vi "PID_controller_09.vi"() -> ()   [LabVIEW 2011]
panel:
  out "x/y":dbl
  out "fit":cluster{"element":dbl, "Value":dbl}[](array[cluster])
  out "err_avg":dbl
  out "Setpoint":string
  out "Angle (deg)":string
  in  "Ks":dbl
  out "dt(s)":dbl
  out "windup error":dbl
  out "tPrev":dbl
  out "target value":dbl
  out "error(t-t0)":cluster{dbl, "Value":dbl}[](array[cluster])
  out "error":dbl
  out "tStart(s)":dbl
  out "S00":dbl
  out "S10":dbl
  out "S20":dbl
  out "S11":dbl
  out "S01":dbl
  out "weight":dbl[](array[numeric])
  in  "# of points to watch":i32
  in  "tSmooth(s)":dbl=-1.0
  out "t0":dbl
  out "error(t)":cluster{dbl, "Value":dbl}[](array[cluster])
  out "error out":errorcluster
  out "first":bool=TRUE
  out "P (torr)":string
  out "XY Graph":T1(graph)
  out "current value":dbl
  in  "stop":bool
  in  "Period (s)":dbl
  out "dValue":dbl
  out "derivative":dbl
  out "integral":dbl
  out "Current angle (deg)":dbl
  in  "Kd":dbl
  in  "Ki":dbl
  in  "Kp":dbl
  out "Current P (torr)":dbl
  in  "Set Point (torr)":dbl
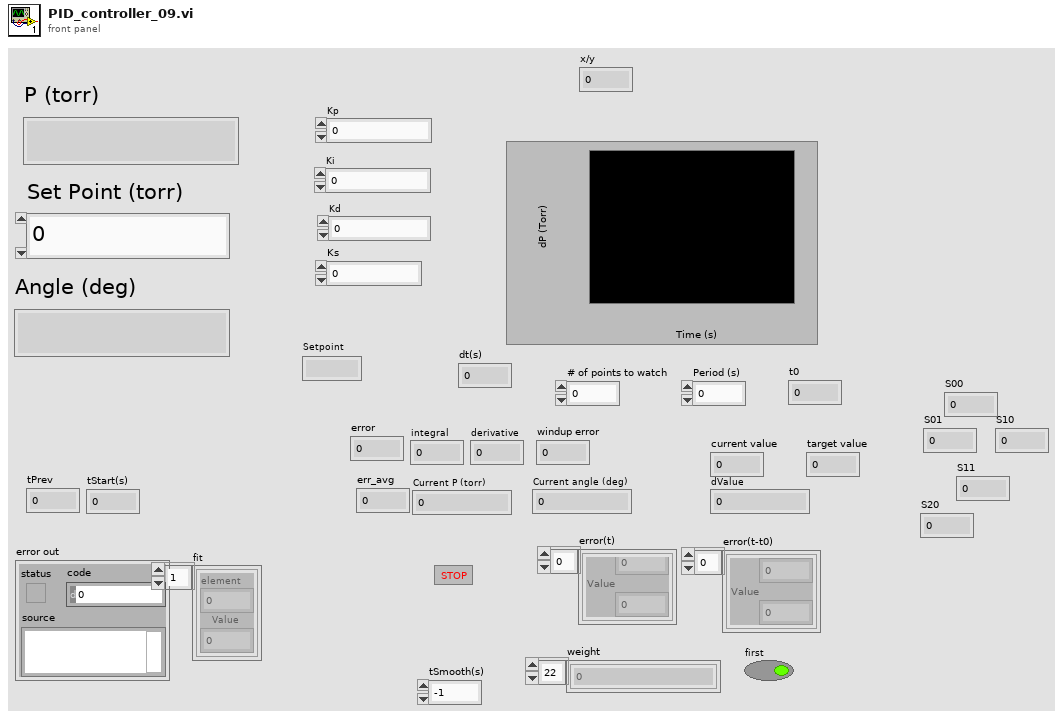
[diagram p1: front panel]
types:
  T1 = cluster{"Value":cluster{"element":dbl, "Value":dbl}[]}[]
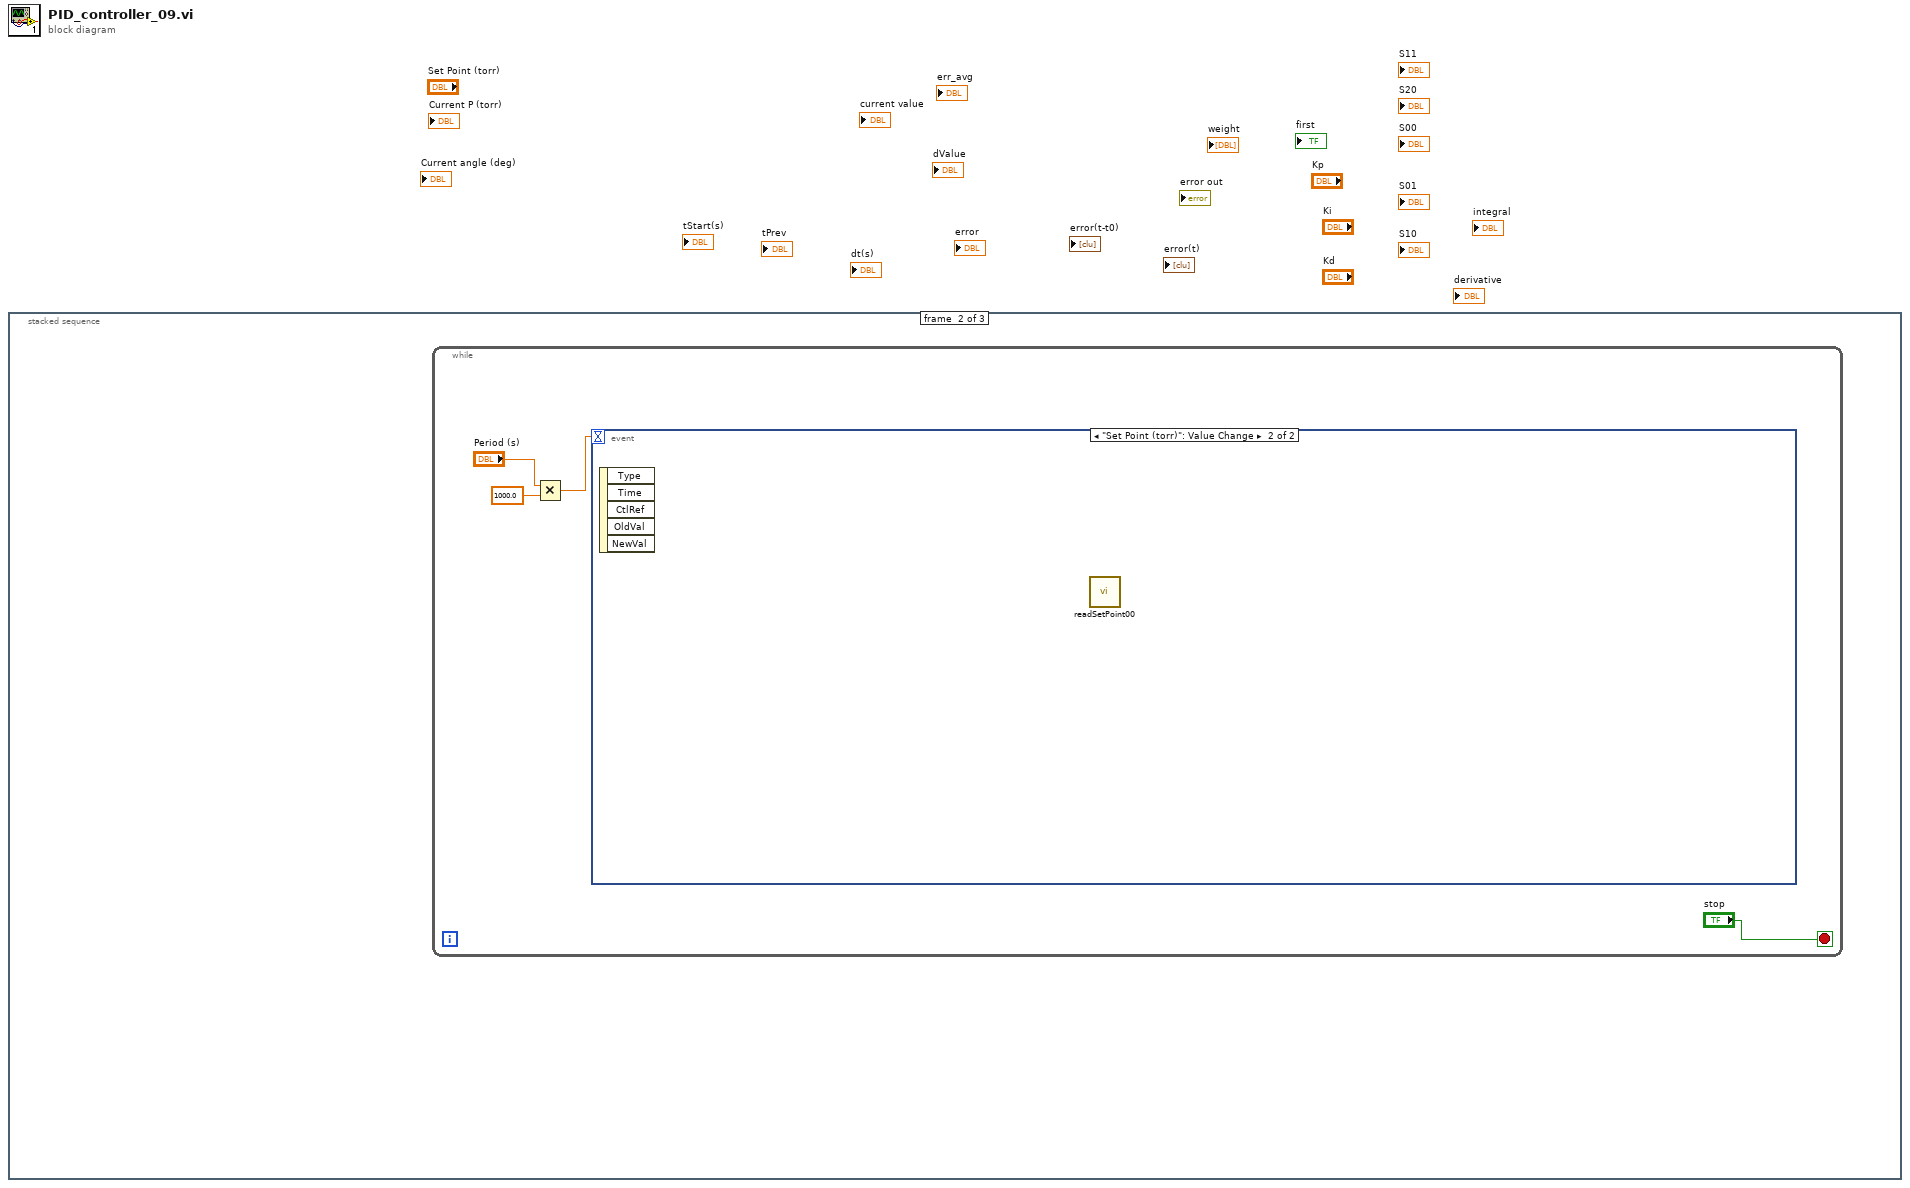
[diagram p0: block diagram]
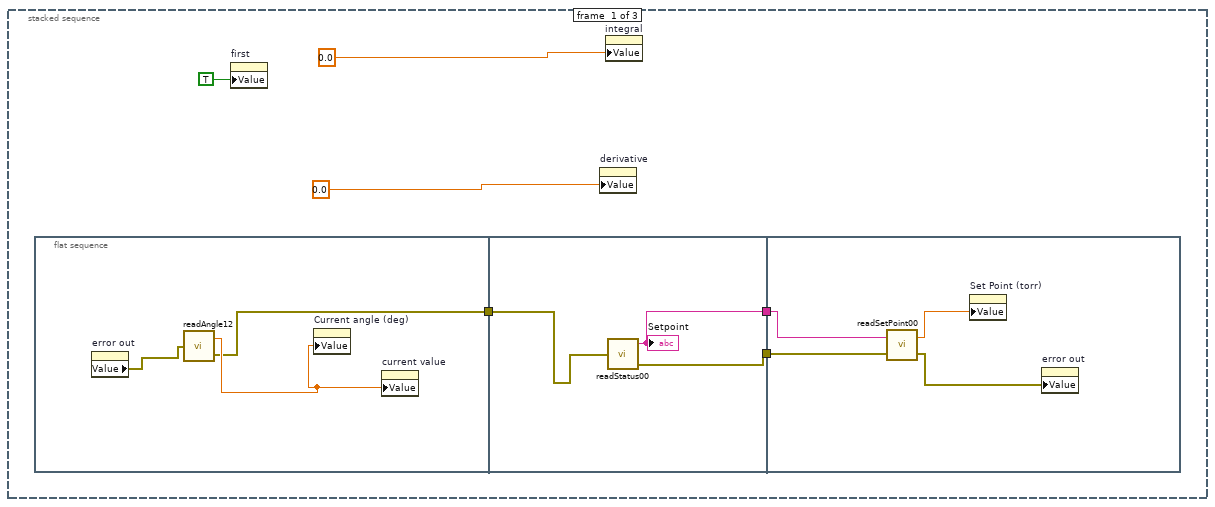
[diagram p2: hidden frame]
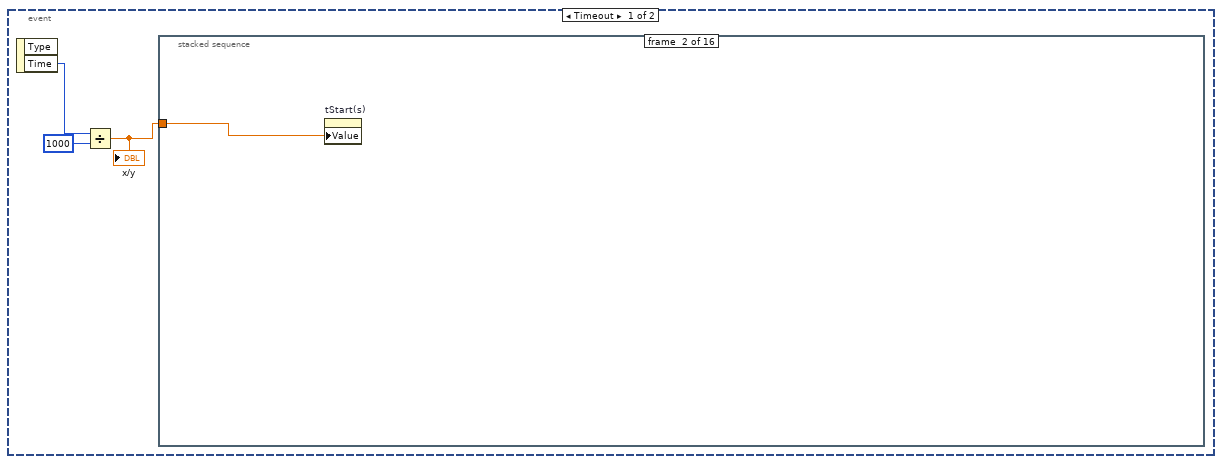
[diagram p3: hidden frame]
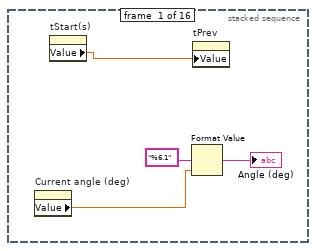
[diagram p4: hidden frame]
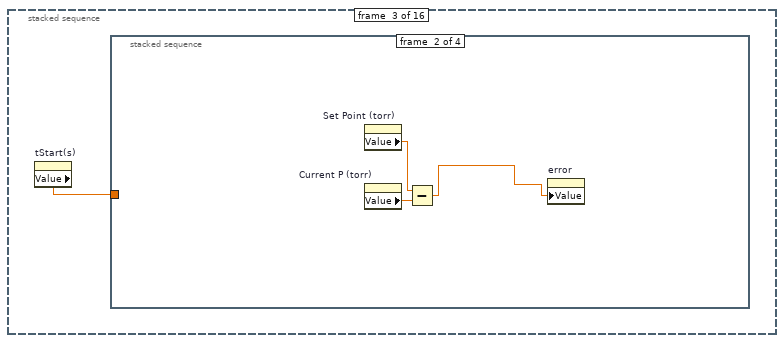
[diagram p5: hidden frame]
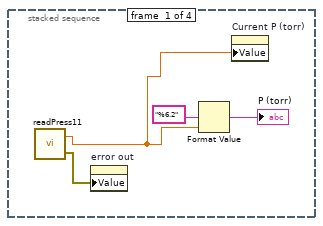
[diagram p6: hidden frame]
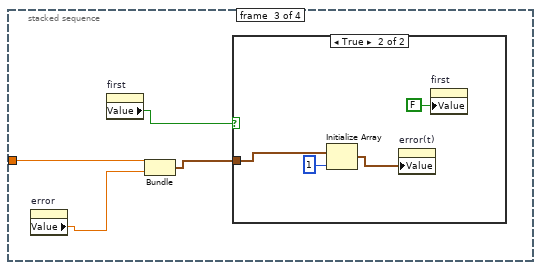
[diagram p7: hidden frame]
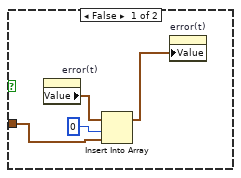
[diagram p8: hidden frame]
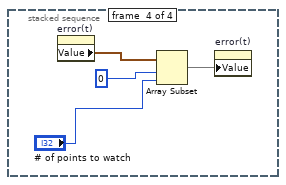
[diagram p9: hidden frame]
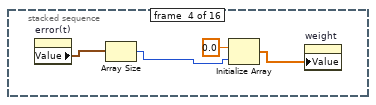
[diagram p10: hidden frame]
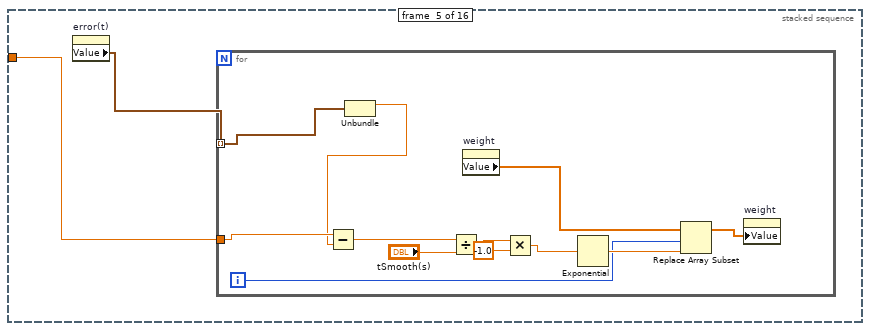
[diagram p11: hidden frame]
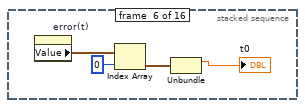
[diagram p12: hidden frame]
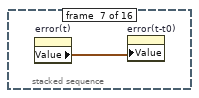
[diagram p13: hidden frame]
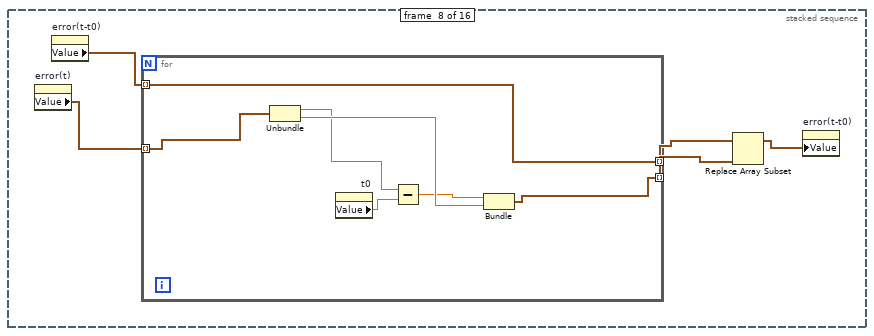
[diagram p14: hidden frame]
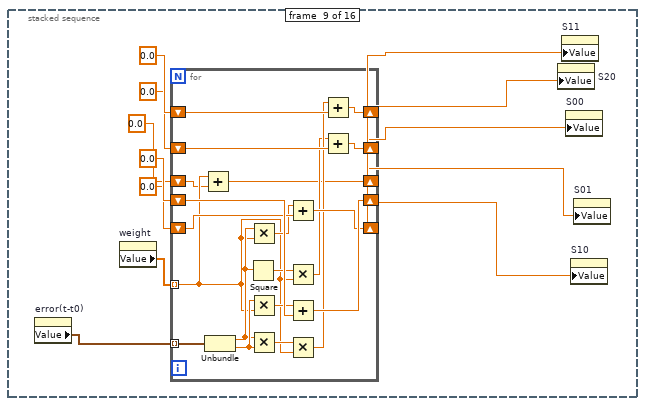
[diagram p15: hidden frame]
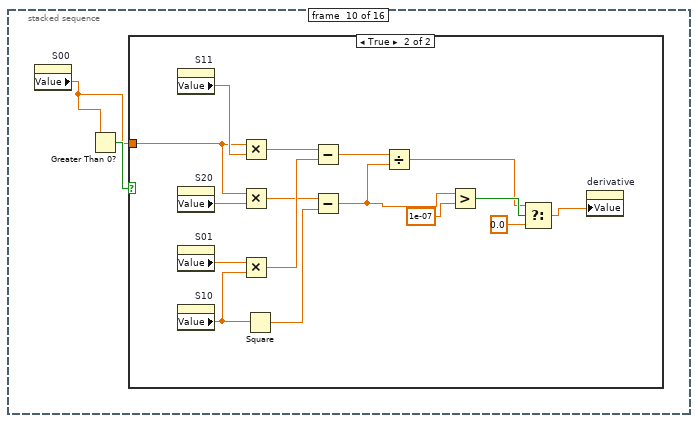
[diagram p16: hidden frame]
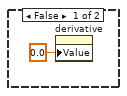
[diagram p17: hidden frame]
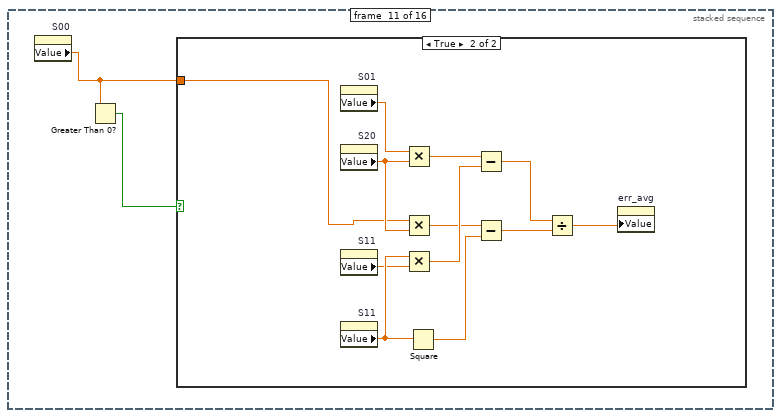
[diagram p18: hidden frame]
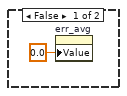
[diagram p19: hidden frame]
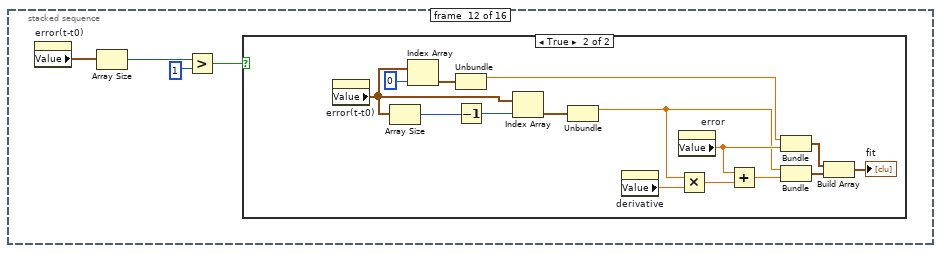
[diagram p20: hidden frame]
diagram:
  n1 = stacked-sequence {
    frame #0 {
      n2 = flat-sequence {
        tunnel: [w7] -> w1
        tunnel: [w12] -> w3
        tunnel: [w11] -> w2
        tunnel: w1 -> [w10]
        tunnel: w3 -> [w16]
        tunnel: w2 -> [w15]
        frame #0 {
          n3 = property on="error out" class="Clust (strict)"() -> ("Value"=w9:errorcluster)  [unwired: 2 in, 2 out]
          n4 = call "readAngle12.vi"("error in"=w9) -> ("angle"=w8:dbl, "error out"=w7:errorcluster)
          n5 = property on="Current angle (deg)" class="DigNum (strict)"("Value"=w8) -> ()  [unwired: 2 in, 2 out]
          n6 = property on="current value" class="DigNum (strict)"("Value"=w8) -> ()  [unwired: 2 in, 2 out]
        }
        frame #1 {
          n7 = call "readStatus00.vi"("error in"=w10) -> ("Setpoint"=w12:string, "error out"=w11:errorcluster)  [unwired: 1 out]
          "Setpoint" <- w12
        }
        frame #2 {
          n8 = call "readSetPoint00.vi"("error in"=w15, "Setpoint"=w16) -> ("error out"=w14:errorcluster, "P"=w13:dbl)
          n9 = property on="Set Point (torr)" class="DigNum (strict)"("Value"=w13) -> ()  [unwired: 2 in, 2 out]
          n10 = property on="error out" class="Clust (strict)"("Value"=w14) -> ()  [unwired: 2 in, 2 out]
        }
      }
      n11 = property on="first" class="Bool (strict)"("Value"=TRUE ("first")) -> ()  [unwired: 2 in, 2 out]
      n12 = property on="derivative" class="DigNum (strict)"("Value"=0.0 ("derivative")) -> ()  [unwired: 2 in, 2 out]
      n13 = property on="integral" class="DigNum (strict)"("Value"=0.0 ("integral")) -> ()  [unwired: 2 in, 2 out]
    }
    frame #1 {
      n14 = while {
        stop <- "stop" stop-if-true
        n15 = Multiply(x="Period (s)", y=1000.0) -> (x*y=w18:dbl)
        n16 = event shown="[1] \"Set Point (torr)\": Value Change" {
          selector: _ -> [_ _]
          dyn-events: _ -> [_ _]
          timeout: w18 -> [_ _]
          event Timeout {
            n17 = event-data() -> ("Time"=w23:u32)  [unwired: 1 in, 1 out]
            n18 = Divide(x=w23, y=u32 1000) -> (x/y=w21:dbl)
            "x/y" <- w21
            n19 = stacked-sequence {
              tunnel: w21 -> [_ w28 _ _ w57 _ _ _ _ _ _ _ _ _ _ _]
              frame #0 {
                n20 = property on="Current angle (deg)" class="DigNum (strict)"() -> ("Value"=w24:dbl)  [unwired: 2 in, 2 out]
                n21 = property on="tStart(s)" class="DigNum (strict)"() -> ("Value"=w27:dbl)  [unwired: 2 in, 2 out]
                n22 = Format Value(format string="%6.1", value (0)=w24) -> (output string=→"Angle (deg)":string)  [unwired: 1 in]
                n23 = property on="tPrev" class="DigNum (strict)"("Value"=w27) -> ()  [unwired: 2 in, 2 out]
              }
              frame #1 {
                n24 = property on="tStart(s)" class="DigNum (strict)"("Value"=w28) -> ()  [unwired: 2 in, 2 out]
              }
              frame #2 {
                n25 = property on="tStart(s)" class="DigNum (strict)"() -> ("Value"=w29:dbl)  [unwired: 2 in, 2 out]
                n26 = stacked-sequence {
                  tunnel: w29 -> [_ _ w39 _]
                  frame #0 {
                    n27 = call "readPress11.vi"() -> ("P"=w31:dbl, "error out"=w30:errorcluster)  [unwired: 1 in]
                    n28 = property on="error out" class="Clust (strict)"("Value"=w30) -> ()  [unwired: 2 in, 2 out]
                    n29 = Format Value(format string="%6.2", value (0)=w31) -> (output string=→"P (torr)":string)  [unwired: 1 in]
                    n30 = property on="Current P (torr)" class="DigNum (strict)"("Value"=w31) -> ()  [unwired: 2 in, 2 out]
                  }
                  frame #1 {
                    n31 = property on="Set Point (torr)" class="DigNum (strict)"() -> ("Value"=w35:dbl)  [unwired: 2 in, 2 out]
                    n32 = property on="Current P (torr)" class="DigNum (strict)"() -> ("Value"=w36:dbl)  [unwired: 2 in, 2 out]
                    n33 = Subtract(x=w35, y=w36) -> (x-y=w34:dbl)
                    n34 = property on="error" class="DigNum (strict)"("Value"=w34) -> ()  [unwired: 2 in, 2 out]
                  }
                  frame #2 {
                    n35 = property on="error" class="DigNum (strict)"() -> ("Value"=w37:dbl)  [unwired: 2 in, 2 out]
                    n36 = property on="first" class="Bool (strict)"() -> ("Value"=w40:bool)  [unwired: 2 in, 2 out]
                    n37 = Bundle("Value"=w39, "Value"=w37) -> (w38:cluster{"Value":dbl, "Value":dbl})  [unwired: 1 in]
                    n38 = case shown="True" w40 {
                      tunnel: w38 -> [w42 w47]
                      frame False {
                        n39 = property on="error(t)" class="Arr (strict)"() -> ("Value"=w43:cluster{dbl, "Value":dbl}[])  [unwired: 2 in, 2 out]
                        n40 = Insert Into Array(array=w43, index=0, new element=w42) -> (w41:cluster{dbl, "Value":dbl}[])
                        n41 = property on="error(t)" class="Arr (strict)"("Value"=w41) -> ()  [unwired: 2 in, 2 out]
                      }
                      frame True {
                        n42 = Initialize Array(w47, 1 ("dimension size")) -> (w45:cluster{"Value":dbl, "Value":dbl}[])
                        n43 = property on="error(t)" class="Arr (strict)"("Value"=w45) -> ()  [unwired: 2 in, 2 out]
                        n44 = property on="first" class="Bool (strict)"("Value"=FALSE ("first")) -> ()  [unwired: 2 in, 2 out]
                      }
                    }
                  }
                  frame #3 {
                    n45 = property on="error(t)" class="Arr (strict)"() -> ("Value"=w50:cluster{dbl, "Value":dbl}[])  [unwired: 2 in, 2 out]
                    n46 = Array Subset(array=w50, index=0, length="# of points to watch") -> (w52:cluster{dbl, "Value":dbl}[])
                    n47 = property on="error(t)" class="Arr (strict)"("Value"=w52) -> ()  [unwired: 2 in, 2 out]
                  }
                }
              }
              frame #3 {
                n48 = property on="error(t)" class="Arr (strict)"() -> ("Value"=w56:cluster{dbl, "Value":dbl}[])  [unwired: 2 in, 2 out]
                n49 = Array Size(array=w56) -> (size(s)=w54:i32)
                n50 = Initialize Array(0.0 ("element"), w54) -> (w53:dbl[])
                n51 = property on="weight" class="Arr (strict)"("Value"=w53) -> ()  [unwired: 2 in, 2 out]
              }
              frame #4 {
                n52 = property on="error(t)" class="Arr (strict)"() -> ("Value"=w58:cluster{dbl, "Value":dbl}[])  [unwired: 2 in, 2 out]
                n53 = for {
                  tunnel: w58 -> [w70] mode=indexing
                  tunnel: w57 -> [w69]
                  i -> [w65]
                  n54 = Unbundle(w70) -> (w68:dbl)  [unwired: 1 out]
                  n55 = Subtract(x=w69, y=w68) -> (x-y=w63:dbl)
                  n56 = Divide(x=w63, y="tSmooth(s)") -> (x/y=w61:dbl)
                  n57 = property on="weight" class="Arr (strict)"() -> ("Value"=w66:dbl[])  [unwired: 2 in, 2 out]
                  n58 = Multiply(x=w61, y=-1.0) -> (x*y=w59:dbl)
                  n59 = Exponential(1:w59) -> (0:w67:dbl)
                  n60 = Replace Array Subset(array=w66, new element=w67, index=w65) -> (w64:dbl[])
                  n61 = property on="weight" class="Arr (strict)"("Value"=w64) -> ()  [unwired: 2 in, 2 out]
                }
              }
              frame #5 {
                n62 = property on="error(t)" class="Arr (strict)"() -> ("Value"=w74:cluster{dbl, "Value":dbl}[])  [unwired: 2 in, 2 out]
                n63 = Index Array(array=w74, index=0) -> (element=w72:cluster{dbl, "Value":dbl})
                n64 = Unbundle(w72) -> (→"t0":dbl)  [unwired: 1 out]
              }
              frame #6 {
                n65 = property on="error(t)" class="Arr (strict)"() -> ("Value"=w75:cluster{dbl, "Value":dbl}[])  [unwired: 2 in, 2 out]
                n66 = property on="error(t-t0)" class="Arr (strict)"("Value"=w75) -> ()  [unwired: 2 in, 2 out]
              }
              frame #7 {
                n67 = property on="error(t)" class="Arr (strict)"() -> ("Value"=w80:cluster{dbl, "Value":dbl}[])  [unwired: 2 in, 2 out]
                n68 = property on="error(t-t0)" class="Arr (strict)"() -> ("Value"=w78:cluster{dbl, "Value":dbl}[])  [unwired: 2 in, 2 out]
                n69 = for {
                  tunnel: w80 -> [w83] mode=indexing
                  tunnel: [w82] -> w79 mode=indexing
                  tunnel: w78 -> [w81] mode=indexing
                  tunnel: [w81] -> w77 mode=indexing
                  n70 = Unbundle(w83) -> (w84:dbl, "Value"=w86:dbl)
                  n71 = property on="t0" class="DigNum (strict)"() -> ("Value"=w87:dbl)  [unwired: 2 in, 2 out]
                  n72 = Subtract(x=w84, y=w87) -> (x-y=w85:dbl)
                  n73 = Bundle(w85, "Value"=w86) -> (w82:cluster{dbl, "Value":dbl})  [unwired: 1 in]
                }
                n74 = Replace Array Subset(array=w77, new element=w79) -> (w76:cluster{dbl, "Value":dbl}[])  [unwired: 1 in]
                n75 = property on="error(t-t0)" class="Arr (strict)"("Value"=w76) -> ()  [unwired: 2 in, 2 out]
              }
              frame #8 {
                n76 = property on="error(t-t0)" class="Arr (strict)"() -> ("Value"=w88:cluster{dbl, "Value":dbl}[])  [unwired: 2 in, 2 out]
                n77 = property on="weight" class="Arr (strict)"() -> ("Value"=w95:dbl[])  [unwired: 2 in, 2 out]
                n78 = for {
                  tunnel: w88 -> [w115] mode=indexing
                  shift-right: [w116] -> w90
                  shift-left: 0.0 -> [w119]
                  shift-right: [w112] -> w93
                  shift-left: 0.0 -> [w118]
                  shift-right: [w111] -> w92
                  shift-left: 0.0 -> [w117]
                  shift-right: [w113] -> w89
                  shift-left: 0.0 -> [w114]
                  tunnel: w95 -> [w102] mode=indexing
                  shift-right: [w100] -> w91
                  shift-left: 0.0 -> [w101]
                  n79 = Add(x=w102, y=w101) -> (x+y=w100:dbl)
                  n80 = Unbundle(w115) -> (w104:dbl, "Value"=w110:dbl)
                  n81 = Square(x=w104) -> (x^2=w106:dbl)
                  n82 = Multiply(x=w104, y=w102) -> (x*y=w103:dbl)
                  n83 = Multiply(x=w110, y=w102) -> (x*y=w109:dbl)
                  n84 = Multiply(x=w104, y=w110) -> (x*y=w108:dbl)
                  n85 = Add(x=w103, y=w114) -> (x+y=w113:dbl)
                  n86 = Multiply(x=w106, y=w102) -> (x*y=w105:dbl)
                  n87 = Add(x=w109, y=w119) -> (x+y=w116:dbl)
                  n88 = Multiply(x=w108, y=w102) -> (x*y=w107:dbl)
                  n89 = Add(x=w107, y=w118) -> (x+y=w112:dbl)
                  n90 = Add(x=w105, y=w117) -> (x+y=w111:dbl)
                }
                n91 = property on="S20" class="DigNum (strict)"("Value"=w92) -> ()  [unwired: 2 in, 2 out]
                n92 = property on="S11" class="DigNum (strict)"("Value"=w93) -> ()  [unwired: 2 in, 2 out]
                n93 = property on="S00" class="DigNum (strict)"("Value"=w91) -> ()  [unwired: 2 in, 2 out]
                n94 = property on="S10" class="DigNum (strict)"("Value"=w89) -> ()  [unwired: 2 in, 2 out]
                n95 = property on="S01" class="DigNum (strict)"("Value"=w90) -> ()  [unwired: 2 in, 2 out]
              }
              frame #9 {
                n96 = property on="S00" class="DigNum (strict)"() -> ("Value"=w120:dbl)  [unwired: 2 in, 2 out]
                n97 = Greater Than 0?(x=w120) -> (x > 0?=w121:bool)
                n98 = case shown="True" w121 {
                  tunnel: w120 -> [_ w130]
                  frame False {
                    n99 = property on="derivative" class="DigNum (strict)"("Value"=0.0 ("derivative")) -> ()  [unwired: 2 in, 2 out]
                  }
                  frame True {
                    n100 = property on="S11" class="DigNum (strict)"() -> ("Value"=w132:dbl)  [unwired: 2 in, 2 out]
                    n101 = property on="S20" class="DigNum (strict)"() -> ("Value"=w131:dbl)  [unwired: 2 in, 2 out]
                    n102 = property on="S01" class="DigNum (strict)"() -> ("Value"=w129:dbl)  [unwired: 2 in, 2 out]
                    n103 = property on="S10" class="DigNum (strict)"() -> ("Value"=w133:dbl)  [unwired: 2 in, 2 out]
                    n104 = Multiply(x=w130, y=w132) -> (x*y=w138:dbl)
                    n105 = Multiply(x=w130, y=w131) -> (x*y=w136:dbl)
                    n106 = Multiply(x=w129, y=w133) -> (x*y=w137:dbl)
                    n107 = Square(x=w133) -> (x^2=w135:dbl)
                    n108 = Subtract(x=w138, y=w137) -> (x-y=w134:dbl)
                    n109 = Subtract(x=w136, y=w135) -> (x-y=w128:dbl)
                    n110 = Divide(x=w134, y=w128) -> (x/y=w124:dbl)
                    n111 = Greater?(x=w128, y=1e-07) -> (0:w126:bool)
                    n112 = Select(t=w124, s=w126, f=0.0) -> (s? t:f=w125:dbl)
                    n113 = property on="derivative" class="DigNum (strict)"("Value"=w125) -> ()  [unwired: 2 in, 2 out]
                  }
                }
              }
              frame #10 {
                n114 = property on="S00" class="DigNum (strict)"() -> ("Value"=w139:dbl)  [unwired: 2 in, 2 out]
                n115 = Greater Than 0?(x=w139) -> (x > 0?=w140:bool)
                n116 = case shown="True" w140 {
                  tunnel: w139 -> [_ w143]
                  frame False {
                    n117 = property on="err_avg" class="DigNum (strict)"("Value"=0.0 ("Pavg")) -> ()  [unwired: 2 in, 2 out]
                  }
                  frame True {
                    n118 = property on="S01" class="DigNum (strict)"() -> ("Value"=w144:dbl)  [unwired: 2 in, 2 out]
                    n119 = property on="S20" class="DigNum (strict)"() -> ("Value"=w147:dbl)  [unwired: 2 in, 2 out]
                    n120 = property on="S11" class="DigNum (strict)"() -> ("Value"=w145:dbl)  [unwired: 2 in, 2 out]
                    n121 = property on="S11" class="DigNum (strict)"() -> ("Value"=w146:dbl)  [unwired: 2 in, 2 out]
                    n122 = Multiply(x=w144, y=w147) -> (x*y=w152:dbl)
                    n123 = Multiply(x=w143, y=w147) -> (x*y=w149:dbl)
                    n124 = Multiply(x=w146, y=w145) -> (x*y=w153:dbl)
                    n125 = Square(x=w146) -> (x^2=w150:dbl)
                    n126 = Subtract(x=w152, y=w153) -> (x-y=w148:dbl)
                    n127 = Subtract(x=w149, y=w150) -> (x-y=w151:dbl)
                    n128 = Divide(x=w148, y=w151) -> (x/y=w142:dbl)
                    n129 = property on="err_avg" class="DigNum (strict)"("Value"=w142) -> ()  [unwired: 2 in, 2 out]
                  }
                }
              }
              frame #11 {
                n130 = property on="error(t-t0)" class="Arr (strict)"() -> ("Value"=w157:cluster{dbl, "Value":dbl}[])  [unwired: 2 in, 2 out]
                n131 = Array Size(array=w157) -> (size(s)=w156:i32)
                n132 = Greater?(x=w156, y=1) -> (0:w154:bool)
                n133 = case shown="True" w154 {
                  frame False {
                  }
                  frame True {
                    n134 = property on="error(t-t0)" class="Arr (strict)"() -> ("Value"=w161:cluster{dbl, "Value":dbl}[])  [unwired: 2 in, 2 out]
                    n135 = Array Size(array=w161) -> (size(s)=w171:i32)
                    n136 = Index Array(array=w161, index=0) -> (element=w169:cluster{dbl, "Value":dbl})
                    n137 = Unbundle(w169) -> (w164:dbl)  [unwired: 1 out]
                    n138 = Decrement(x=w171) -> (x-1=w170:i32)
                    n139 = Index Array(array=w161, index=w170) -> (element=w168:cluster{dbl, "Value":dbl})
                    n140 = Unbundle(w168) -> (w162:dbl)  [unwired: 1 out]
                    n141 = property on="derivative" class="DigNum (strict)"() -> ("Value"=w167:dbl)  [unwired: 2 in, 2 out]
                    n142 = property on="error" class="DigNum (strict)"() -> ("Value"=w165:dbl)  [unwired: 2 in, 2 out]
                    n143 = Multiply(x=w162, y=w167) -> (x*y=w166:dbl)
                    n144 = Add(x=w165, y=w166) -> (x+y=w163:dbl)
                    n145 = Bundle(w164, "Value"=w165) -> (w160:cluster{dbl, "Value":dbl})  [unwired: 1 in]
                    n146 = Bundle(w162, w163) -> (w159:cluster{dbl, dbl})  [unwired: 1 in]
                    n147 = Build Array(w160, w159) -> (→"fit":cluster{dbl, "Value":dbl}[])
                  }
                }
              }
              frame #12 {
                n148 = property on="error" class="DigNum (strict)"() -> ("Value"=w177:dbl)  [unwired: 2 in, 2 out]
                n149 = property on="tPrev" class="DigNum (strict)"() -> ("Value"=w178:dbl)  [unwired: 2 in, 2 out]
                n150 = property on="tStart(s)" class="DigNum (strict)"() -> ("Value"=w179:dbl)  [unwired: 2 in, 2 out]
                n151 = Subtract(x=w179, y=w178) -> (x-y=w173:dbl)
                n152 = property on="dt(s)" class="DigNum (strict)"("Value"=w173) -> ()  [unwired: 2 in, 2 out]
                n153 = property on="integral" class="DigNum (strict)"() -> ("Value"=w175:dbl)  [unwired: 2 in, 2 out]
                n154 = Multiply(x=w177, y=w173) -> (x*y=w176:dbl)
                n155 = Add(x=w176, y=w175) -> (x+y=w174:dbl)
                n156 = property on="integral" class="DigNum (strict)"("Value"=w174) -> ()  [unwired: 2 in, 2 out]
              }
              frame #13 {
                n157 = property on="error" class="DigNum (strict)"() -> ("Value"=w180:dbl)  [unwired: 2 in, 2 out]
                n158 = property on="Kp" class="DigNum (strict)"() -> ("Value"=w190:dbl)  [unwired: 2 in, 2 out]
                n159 = property on="integral" class="DigNum (strict)"() -> ("Value"=w188:dbl)  [unwired: 2 in, 2 out]
                n160 = property on="derivative" class="DigNum (strict)"() -> ("Value"=w186:dbl)  [unwired: 2 in, 2 out]
                n161 = property on="Ki" class="DigNum (strict)"() -> ("Value"=w189:dbl)  [unwired: 2 in, 2 out]
                n162 = property on="Kd" class="DigNum (strict)"() -> ("Value"=w187:dbl)  [unwired: 2 in, 2 out]
                n163 = Multiply(x=w187, y=w186) -> (x*y=w183:dbl)
                n164 = Multiply(x=w189, y=w188) -> (x*y=w184:dbl)
                n165 = Multiply(x=w190, y=w180) -> (x*y=w185:dbl)
                n166 = Add(x=w185, y=w184) -> (x+y=w182:dbl)
                n167 = Add(x=w182, y=w183) -> (x+y=w181:dbl)
                n168 = property on="dValue" class="DigNum (strict)"("Value"=w181) -> ()  [unwired: 2 in, 2 out]
              }
              frame #14 {
                w200 = 90.0 ("y")
                n169 = property on="dValue" class="DigNum (strict)"() -> ("Value"=w207:dbl)  [unwired: 2 in, 2 out]
                n170 = property on="current value" class="DigNum (strict)"() -> ("Value"=w208:dbl)  [unwired: 2 in, 2 out]
                n171 = Add(x=w208, y=w207) -> (x+y=w191:dbl)
                "target value" <- w191
                n172 = Less Than 0?(x=w191) -> (x < 0?=w204:bool)
                n173 = Select(t=0.0, s=w204, f=w191) -> (s? t:f=w201:dbl)
                n174 = property on="error out" class="Clust (strict)"() -> ("Value"=w206:errorcluster)  [unwired: 2 in, 2 out]
                n175 = Greater?(x=w201, y=w200) -> (0:w202:bool)
                n176 = Select(t=w200, s=w202, f=w201) -> (s? t:f=w192:dbl)
                n177 = Subtract(x=w192, y=w191) -> (x-y=w199:dbl)
                "windup error" <- w199
                n178 = call "setAngle_00.vi"("error in (no error)"=w206, "Angle (deg)"=w192) -> ("error out"=w205:errorcluster)
                n179 = property on="Current angle (deg)" class="DigNum (strict)"("Value"=w192) -> ()  [unwired: 2 in, 2 out]
                n180 = property on="dt(s)" class="DigNum (strict)"() -> ("Value"=w198:dbl)  [unwired: 2 in, 2 out]
                n181 = property on="current value" class="DigNum (strict)"("Value"=w192) -> ()  [unwired: 2 in, 2 out]
                n182 = property on="error out" class="Clust (strict)"("Value"=w205) -> ()  [unwired: 2 in, 2 out]
                n183 = Multiply(x=w199, y=w198) -> (x*y=w197:dbl)
                n184 = property on="integral" class="DigNum (strict)"() -> ("Value"=w194:dbl)  [unwired: 2 in, 2 out]
                n185 = Multiply(x="Ks", y=w197) -> (x*y=w195:dbl)
                n186 = Add(x=w195, y=w194) -> (x+y=w193:dbl)
                n187 = property on="integral" class="DigNum (strict)"("Value"=w193) -> ()  [unwired: 2 in, 2 out]
              }
              frame #15 {
                n188 = property on="fit" class="Arr (strict)"() -> ("Value"=w211:cluster{"element":dbl, "Value":dbl}[])  [unwired: 2 in, 2 out]
                n189 = property on="error(t-t0)" class="Arr (strict)"() -> ("Value"=w210:cluster{dbl, "Value":dbl}[])  [unwired: 2 in, 2 out]
                n190 = Build Cluster Array(w210, w211) -> (→"XY Graph":T1)
              }
            }
          }
          event "Set Point (torr)": Value Change {
            n191 = event-data() -> ()  [unwired: 1 in, 5 out]
            n192 = call "readSetPoint00.vi"() -> ()  [unwired: 2 in, 2 out]
          }
        }
      }
    }
    frame #2 {
      n193 = flat-sequence {
        frame #0 {
          n194 = call "WriteAdaptorr03.vi"("string to write"="D5") -> ()  [unwired: 1 in, 1 out]
        }
        frame #1 {
          n195 = property on="Setpoint" class="Str"() -> ("Value"=w214:string)  [unwired: 2 in, 2 out]
          n196 = Concatenate Strings("Press ", w214, " on AdapTorr") -> (w213:string)
          n197 = One Button Dialog(message=w213) -> ()  [unwired: 1 in, 1 out]
        }
      }
    }
  }
